vi "Destroy Session Reservations.vi"(8 "error in":errorcluster, 11 "measurement context in":refnum<class "MeasurementContext.lvclass">) -> (0 "error out":errorcluster, 3 "measurement context out":refnum<class "MeasurementContext.lvclass">)   [LabVIEW 2020, in "MeasurementLink Measurement Server.lvlib" / "MeasurementContext.lvclass"]
uses:
  MeasurementContext.lvclass
  MeasurementContext.lvclass/MeasurementContext.ctl
  MeasurementLink Session Management/Session Reservation/Session Reservation.lvclass
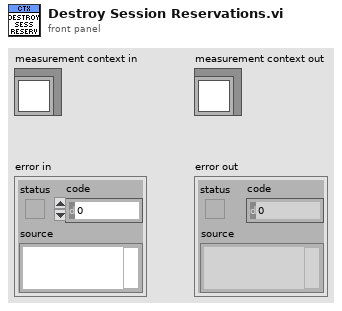
[diagram p1: front panel]
types:
  T1 = typedef "MeasurementLink Measurement Server.lvlib/MeasurementContext.lvclass/Data.ctl" = cluster{"PinMapContext":T2, "gRPCServerId":T3, "IMeasurementService":refnum<class "IMeasurementService.lvclass">, "MeasurementPluginService":refnum<class "MeasurementPluginService.lvclass">, "Session Reservations":refnum<class "Session Reservation.lvclass">[]}
  T2 = typedef "MeasurementLink Measurement Server.lvlib/PinMapContext.ctl" = cluster{"pin_map_id":string, "sites":i32[]}
  T3 = typedef "grpc-lvsupport-release.lvlib/grpcId.ctl" = u64
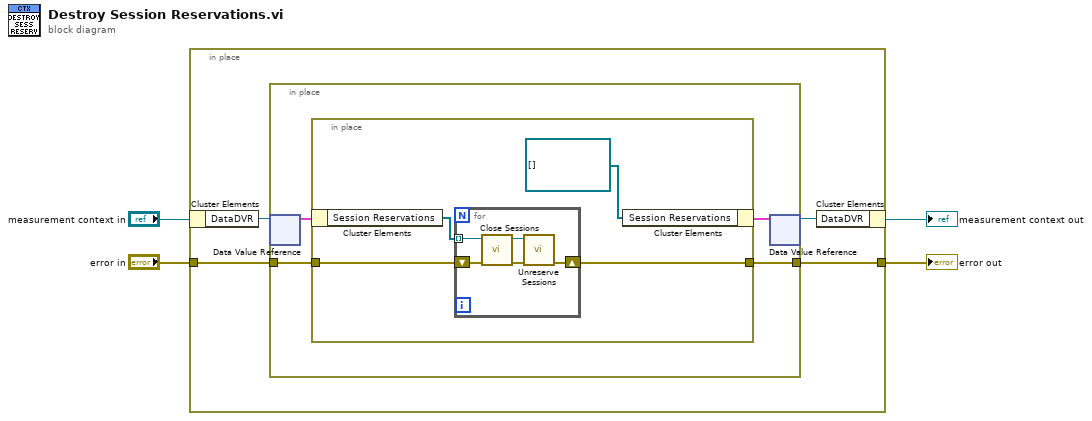
[diagram p0: block diagram]
diagram:
  n1 = in-place {
    in-place-border: "error in" -> [w6]
    in-place-border: [w5] -> w3
    n2 = in-place-cluster #1("measurement context in") -> ("DataDVR"=w8:refnum<data-value>)
    n3 = in-place {
      in-place-border: w6 -> [w10]
      in-place-border: [w9] -> w5
      n4 = in-place-dvr #2(w8) -> (w12:T1)  [unwired: 1 out]
      n5 = in-place {
        in-place-border: w10 -> [w14]
        in-place-border: [w13] -> w9
        n6 = in-place-cluster #3(w12) -> ("Session Reservations"=w15:refnum<class "Session Reservation.lvclass">[])
        n7 = for {
          tunnel: w15 -> [w21] mode=indexing
          shift-right: [w20] -> w13
          shift-left: w14 -> [w18]
          n8 = call "Close Sessions.vi"("error in"=w18, "session reservation in"=w21) -> ("error out"=w17:errorcluster, "session reservation out"=w19:refnum<class "Session Reservation.lvclass">)  [unwired: 8 in]
          n9 = call "Unreserve Sessions.vi"("error in"=w17, "session reservation in"=w19) -> ("error out"=w20:errorcluster)  [unwired: 9 in]
        }
        n10 = in-place-cluster #3("Session Reservations"=refnum<class "Session Reservation.lvclass">[] []) -> (w11:T1)
      }
      n11 = in-place-dvr #2(w11) -> (w7:refnum<data-value>)  [unwired: 1 out]
    }
    n12 = in-place-cluster #1("DataDVR"=w7) -> (→"measurement context out":refnum<class "MeasurementContext.lvclass">)
  }
  "error out" <- w3
